vi "openXMLFile.vi"(8 "error in (no error)":errorcluster, 10 "Path":path, 11 "XmlParser in":refnum<class "XmlParser.lvclass">) -> (0 "error out":errorcluster, 1 "xmlFileInput":string, 3 "XmlParser out":refnum<class "XmlParser.lvclass">)   [LabVIEW 2011, in "Tools.lvlib" / "xml.lvlib" / "XmlParser.lvclass"]
doc: "Open xml document from Path and read it to a string.\nShould be used the readInxml which will make that string an xml node."
uses:
  XmlParser.lvclass
  XmlParser.lvclass/XmlParser.ctl
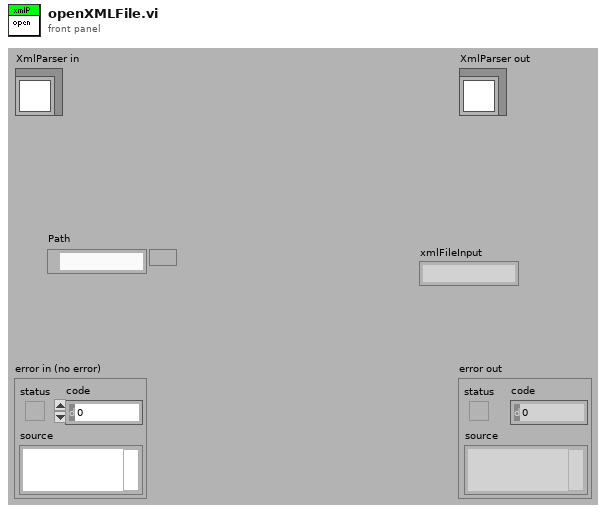
[diagram p1: front panel]
types:
  T1 = enum16{"open", "replace", "create", "open or create", "replace or create", "replace or create with confirmation"}
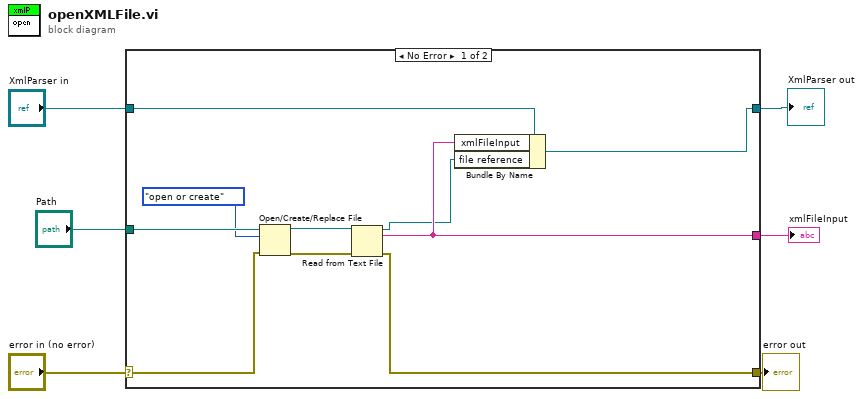
[diagram p0: block diagram]
diagram:
  n1 = case shown="No Error" "error in (no error)" {
    selector: "error in (no error)" -> [w15 w18]
    tunnel: [w12 w18] -> w5
    tunnel: [w10 w17] -> w3
    tunnel: "XmlParser in" -> [w11 w17]
    tunnel: "Path" -> [w16 _]
    tunnel: [w9 _] -> w1
    frame No Error {
      n2 = Open/Create/Replace File(file path (use dialog)=w16, error in=w15, operation (0:open)=T1."open or create") -> (refnum out=w14:refnum<file>, error out=w13:errorcluster)  [unwired: 3 in, 1 out]
      n3 = Read from Text File(file (use dialog)=w14, error in=w13) -> (refnum out=w8:refnum<file>, text=w9:string, error out=w12:errorcluster)  [unwired: 2 in, 1 out]
      n4 = Bundle By Name(cluster=w11, "xmlFileInput"=w9, "file reference"=w8) -> (w10:refnum<class "XmlParser.lvclass">)
    }
    frame Error {
    }
  }
  "error out" <- w5
  "XmlParser out" <- w3
  "xmlFileInput" <- w1
